vi "Matrix_ExtractCol_To_1D_Array.vi"(9 "Column index":i32, 11 "Input Matrix":T1) -> (3 "Column Array":dbl[](array[numeric]))   [LabVIEW 2019]
uses:
  <vilib>/Analysis/Matrix/NI_Matrix.lvlib
  <vilib>/Analysis/Matrix/Numeric/Conversions/Matrix To Array - RM.vi
  <vilib>/Analysis/Matrix/Datatypes/RealMatrix.ctl
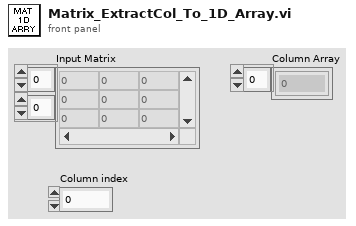
[diagram p1: front panel]
types:
  T1 = typedef "NI_Matrix.lvlib/RealMatrix.ctl" = dbl[][]
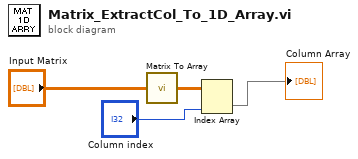
[diagram p0: block diagram]
diagram:
  n1 = call-poly <vilib>:"Matrix To Array.vi"("Real Matrix"="Input Matrix") -> ("Real 2D Array"=w2:dbl[][])
  n2 = Index Array(array=w2, index (col)="Column index") -> (element=→"Column Array":dbl[])  [unwired: 1 in]
